vi "Timout_Operations.vi"(7 "PosIn":dbl[](array[numeric]), 8 "error in":errorcluster caption="error out", 9 "Connected?":bool, 10 "NumberOfAxes":u8, 11 "plLSID":i32) -> (0 "error out":errorcluster, 1 "AnaOut2":i32, 2 "Anaout1":i32, 3 "LimitsOutput":T1[](array[typedef]), 5 "PosOut":dbl[](array[numeric]))   [LabVIEW 2018]
uses:
  Axis_Switch.ctl
  <userlib>/TANGO_DLL/Tango_DLL.lvlib
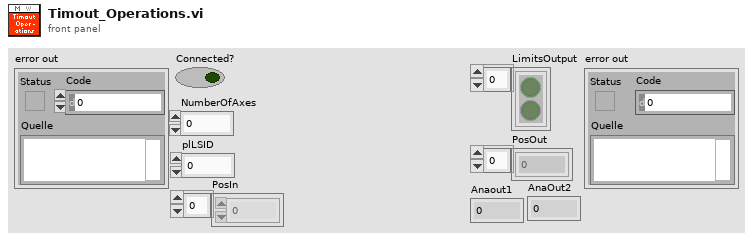
[diagram p1: front panel]
types:
  T1 = typedef "Axis_Switch.ctl" = cluster{"E0":bool, "EE":bool}
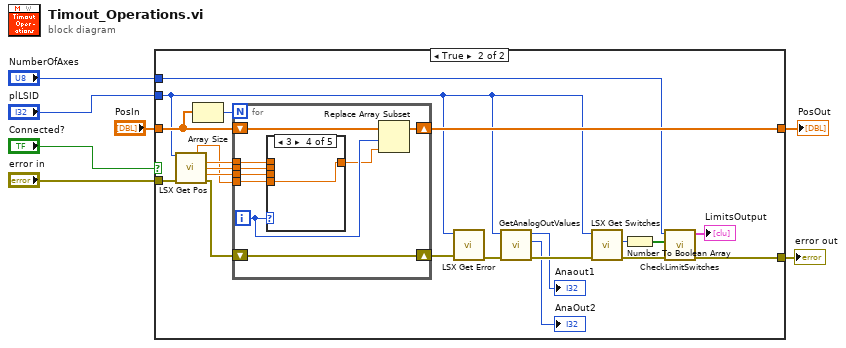
[diagram p0: block diagram]
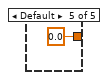
[diagram p6: hidden frame]
diagram:
  n1 = case shown="True" "Connected?" {
    tunnel: "error in" -> [w9 w30]
    tunnel: "PosIn" -> [w8 w28]
    tunnel: [w9 w17] -> w1
    tunnel: "plLSID" -> [_ w14]
    tunnel: [w8 w27] -> w2
    tunnel: "NumberOfAxes" -> [_ w19]
    frame False {
    }
    frame True {
      n2 = call <userlib>:"LSX Get Pos.vi"("lLSID"=w14, "error in (no error)"=w30) -> ("pdA out"=w23:dbl, "pdX out"=w26:dbl, "pdY out"=w25:dbl, "pdZ out"=w24:dbl, "error out"=w11:errorcluster)  [unwired: 8 in, 1 out]
      n3 = Array Size(array=w28) -> (size(s)=w29:i32)
      n4 = for {
        N: w29 -> [_]
        tunnel: w26 -> [w38]
        tunnel: w25 -> [w37]
        tunnel: w24 -> [w36]
        tunnel: w23 -> [w35]
        shift-right: [w32] -> w27
        shift-left: w28 -> [w39]
        shift-right: [w31] -> w10
        shift-left: w11 -> [w31]
        i -> [w34]
        n5 = case shown="3" w34 {
          tunnel: w38 -> [w40 _ _ _ _]
          tunnel: w37 -> [_ w41 _ _ _]
          tunnel: w36 -> [_ _ w42 _ _]
          tunnel: w35 -> [_ _ _ w43 _]
          tunnel: [w40 w41 w42 w43 0.0 ("pdA out")] -> w33
          frame 0 {
          }
          frame 1 {
          }
          frame 2 {
          }
          frame 3 {
          }
          frame Default {
          }
        }
        n6 = Replace Array Subset(array=w39, new element=w33, index=w34) -> (w32:dbl[])
      }
      n7 = call <userlib>:"LSX Get Error.vi"("error in (no error)"=w10, "lLSID"=w14) -> ("error out"=w16:errorcluster)  [unwired: 7 in, 2 out]
      n8 = call "GetAnalogOutValues.vi"("error in (no error)"=w16, "lLSID"=w14) -> ("error out"=w15:errorcluster, "AnaOut2"=→"AnaOut2":i32, "Anaout1"=→"Anaout1":i32)  [unwired: 7 in]
      n9 = call <userlib>:"LSX Get Switches.vi"("error in (no error)"=w15, "lLSID"=w14) -> ("error out"=w20:errorcluster, "plFlags out"=w22:i32)  [unwired: 7 in, 1 out]
      n10 = Number To Boolean Array(number=w22) -> (Boolean array=w21:bool[])
      n11 = call "CheckLimitSwitches.vi"("error in (no error)"=w20, "BoolArrayIn"=w21, "NumberOfAxes"=w19) -> ("error out"=w17:errorcluster, "LimitsOutput"=→"LimitsOutput":T1[])  [unwired: 7 in]
    }
  }
  "PosOut" <- w2
  "error out" <- w1
